vi "H5Oexists_by_name.vi"(6 "lapl_id":T1, 8 "error in (no error)":errorcluster, 10 "Object Name":string, 11 "Location Ref":T1) -> (0 "error out":errorcluster, 2 "Exists":bool, 3 "Location Ref out":T1)   [LabVIEW 2017]
doc: "Determines whether a link resolves to an actual object."
uses:
  <vilib>/UPVI/lvhdf5/library.llb/HDF5 Ref.ctl
  <vilib>/UPVI/lvhdf5/hdf5.dll
panel:
  # "LVHDF5 Toolkit\nCopyright (c) 2005-2013 by Jason D. Sommerville\nCopyright (c) 2014-2015 by UPVI, LLC.\n\nThis use and distribution of this file is governed by the terms found in \nLICENSE.txt distributed with this toolkit and installed at\n <user.lib>\\_lvhdf5\\LICENSE.txt"
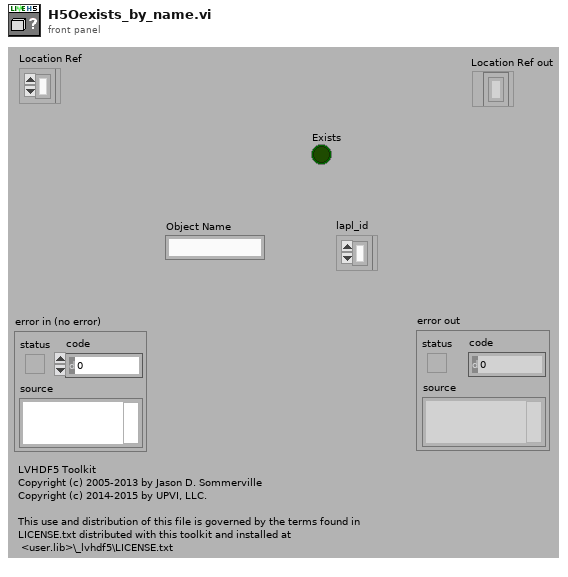
[diagram p1: front panel]
types:
  T1 = typedef "HDF5 Ref.ctl" = refnum<k1>
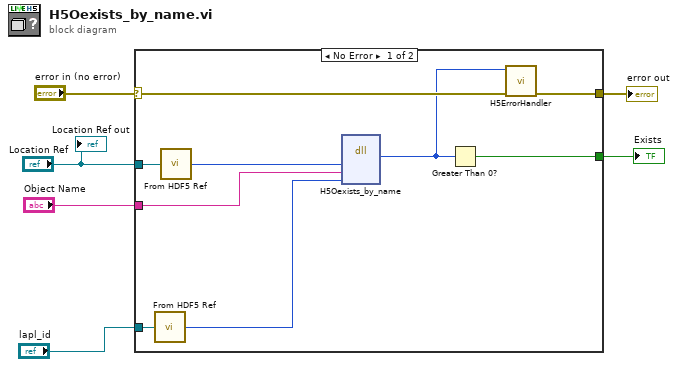
[diagram p0: block diagram]
diagram:
  n1 = case shown="No Error" "error in (no error)" {
    selector: "error in (no error)" -> [w15 w16]
    tunnel: [w14 w16] -> w5
    tunnel: "Location Ref" -> [w13 _]
    tunnel: "Object Name" -> [w7 _]
    tunnel: "lapl_id" -> [w12 _]
    tunnel: [w8 _] -> w1
    frame No Error {
      n2 = call <vilib>:"From HDF5 Ref.vi"("HDF5 Ref"=w12) -> ("I32"=w11:i32)
      n3 = call <vilib>:"From HDF5 Ref.vi"("HDF5 Ref"=w13) -> ("I32"=w10:i32)
      n4 = dll-call lib="C:/Program Files/National Instruments/LabVIEW 2017/vi.lib/UPVI/lvhdf5/hdf5.dll" fn="H5Oexists_by_name"("loc_id"=w10, "name"=w7, "lapl_id"=w11) -> ("return type"=w9:i32)  [unwired: 6 in, 2 out]
      n5 = Greater Than 0?(x=w9) -> (x > 0?=w8:bool)
      n6 = call <vilib>:"H5ErrorHandler.vi"("error in (no error)"=w15, "herr_t"=w9) -> ("error out"=w14:errorcluster)  [unwired: 3 in, 4 out]
    }
    frame Error {
    }
  }
  "error out" <- w5
  "Exists" <- w1
  "Location Ref out" <- "Location Ref"
